vi "Interface_Asset_Write Process Name.vi"(10 "Process Name":string, 11 "AssetInterface in":refnum<class "Interface_Asset.lvclass">) -> (3 "AssetInterface out":refnum<class "Interface_Asset.lvclass">)   [LabVIEW 2015, in "Interface_Asset.lvclass"]
uses:
  Interface_Asset.lvclass
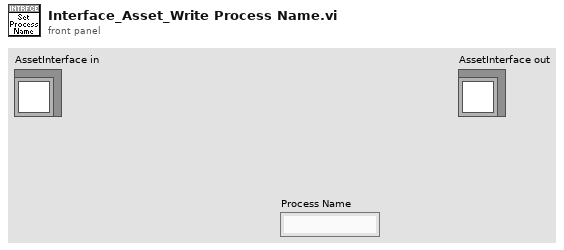
[diagram p1: front panel]
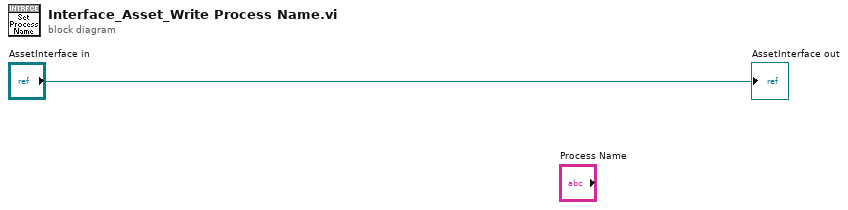
[diagram p0: block diagram]
diagram:
  "AssetInterface out" <- "AssetInterface in"
